vi "obtain controllers test.vi"() -> ()   [LabVIEW 2021, in "Test VIs.lvclass"]
uses:
  Test VIs.lvclass
  Classes/Controller/Controller.lvclass
panel:
  out "Dispenser error?":bool
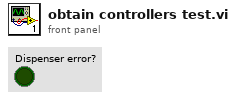
[diagram p1: front panel]
types:
  T1 = typedef "Controller.lvclass/Controllers.ctl" = cluster{"I-O.lvclass":refnum<class "I-O.lvclass">, "Gantry":refnum<k24>, "Dispenser":refnum<visa-resource-name>}
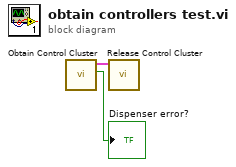
[diagram p0: block diagram]
diagram:
  n1 = call "Obtain Control Cluster.vi"() -> ("Dispenser error?"=→"Dispenser error?":bool, "Control Out"=w2:T1)  [unwired: 10 in]
  n2 = call "Release Control Cluster.vi"("output cluster"=w2) -> ()  [unwired: 11 in]
